vi "Read serial type.vi"(8 "error in (no error)":errorcluster, 11 "Modbus Slave configuration in":refnum<class "Modbus Slave configuration.lvclass">) -> (0 "error out":errorcluster, 2 "serial type":enum16{"RTU", "ASCII"}(ring), 3 "Modbus Slave configuration out":refnum<class "Modbus Slave configuration.lvclass">)   [LabVIEW 2013, in "Modbus Slave configuration.lvclass"]
uses:
  Modbus Slave configuration.lvclass
  Modbus Slave configuration.lvclass/Modbus Slave configuration.ctl
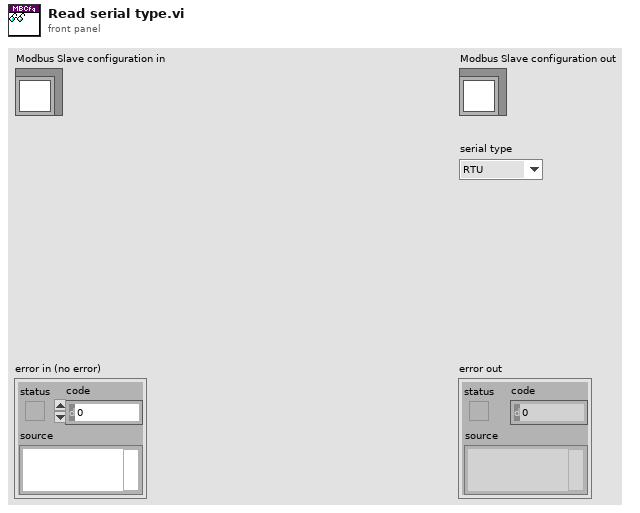
[diagram p1: front panel]
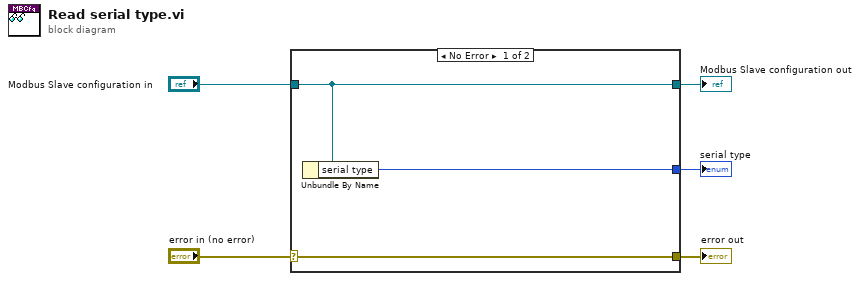
[diagram p0: block diagram]
diagram:
  n1 = case shown="No Error" "error in (no error)" {
    selector: "error in (no error)" -> [w8 w9]
    tunnel: [w8 w9] -> w4
    tunnel: [w7 w10] -> w2
    tunnel: "Modbus Slave configuration in" -> [w7 w10]
    tunnel: [w6 _] -> w1
    frame No Error {
      n2 = Unbundle By Name(w7) -> ("serial type"=w6:enum16{"RTU", "ASCII"})
    }
    frame Error {
    }
  }
  "error out" <- w4
  "Modbus Slave configuration out" <- w2
  "serial type" <- w1
